vi "MessageBase.getFieldValue.vi"(8 "error in (no error)":errorcluster, 10 "FIeld.Name":string="Length", 11 "MessageBase in":refnum<class "MessageBase.lvclass">) -> (0 "error out":errorcluster, 2 "FieldValue":variant, 3 "MessageBase out":refnum<class "MessageBase.lvclass">)   [LabVIEW 2022 SP3, in "MessageBase.lvclass"]
uses:
  MessageBase.lvclass
  MessageBase.lvclass/MessageBase.ctl
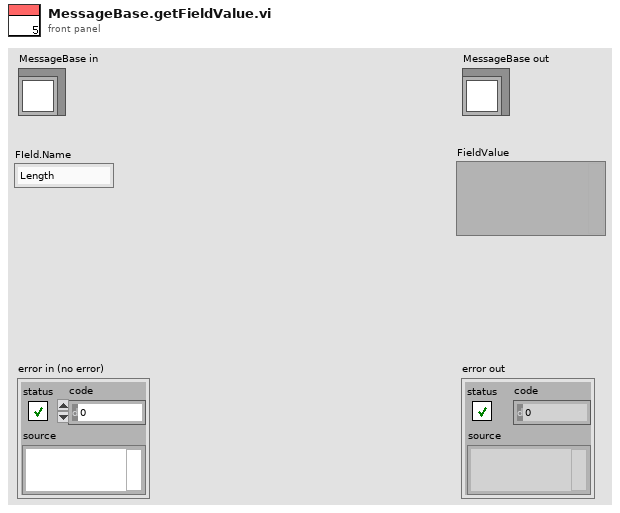
[diagram p1: front panel]
types:
  T1 = typedef "FieldSpec.ctl" = cluster{"Name":string, "Offset":i32, "Length":i32, "FieldType":enum16{"Alphanumeric", "Binary", "BinaryLongPrice", "BinaryShortPrice", "BitField", "PrintableAscii", "Value"}, "FieldValue":variant}
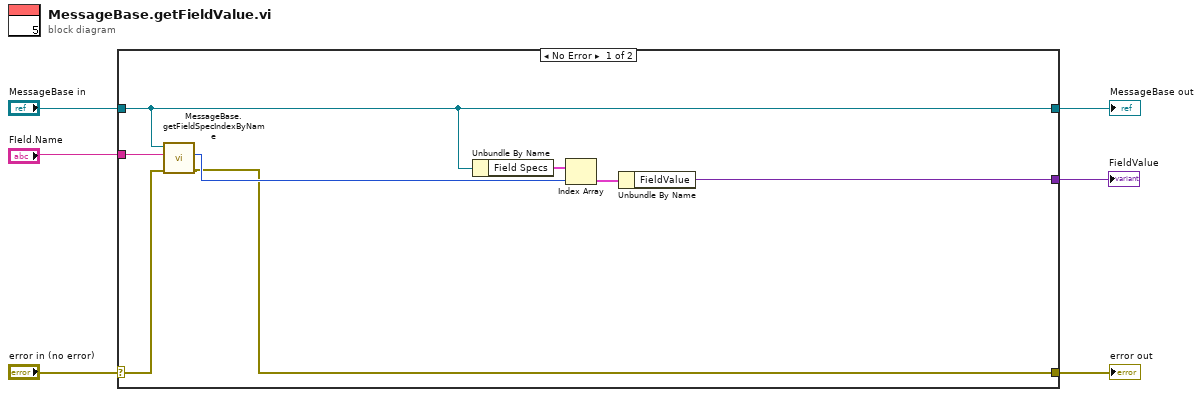
[diagram p0: block diagram]
diagram:
  n1 = case shown="No Error" "error in (no error)" {
    selector: "error in (no error)" -> [w11 w15]
    tunnel: [w10 w15] -> w5
    tunnel: [w7 w16] -> w3
    tunnel: "MessageBase in" -> [w7 w16]
    tunnel: "FIeld.Name" -> [w14 _]
    tunnel: [w8 _] -> w1
    frame No Error {
      n2 = call-dynamic "MessageBase.getFieldSpecIndexByName.vi"("error in (no error)"=w11, "Field.Name"=w14, "MessageBase in"=w7) -> ("error out"=w10:errorcluster, "Index"=w12:i32)  [unwired: 6 in, 1 out]
      n3 = Unbundle By Name(w7) -> ("Field Specs"=w13:T1[])
      n4 = Index Array(array=w13, index=w12) -> (element=w9:T1)
      n5 = Unbundle By Name(w9) -> ("FieldValue"=w8:variant)
    }
    frame Error {
      # "Wire the error cluster across even in the \"No Error\"\ncase so that warnings get propagated."
    }
  }
  "error out" <- w5
  "MessageBase out" <- w3
  "FieldValue" <- w1
